vi "IniEVEScrew.vi"(8 "error in":errorcluster, 10 "Screw section":string="Info", 11 "INI file path":path=path "D:/ZDX201 塗膠螺絲鎖固自動化_鴻海/ZDX201_LabView/iniData/screw_iniData.ini") -> (0 "L_file":string, 1 "R_file":string, 2 "螺絲高度LL":dbl, 3 "螺絲高度UL":dbl, 4 "txt path":path, 5 "自動運行":bool, 6 "分析計算時間":u32, 7 "offset":dbl=2.4009)   [LabVIEW 2019]
uses:
  <vilib>/Utility/config.llb/Read Key (Double).vi
  <vilib>/Utility/config.llb/Read Key (Path).vi
  <vilib>/Utility/config.llb/Read Key (String).vi
  <vilib>/Utility/config.llb/Read Key (Boolean).vi
  <vilib>/Utility/config.llb/Read Key (U32).vi
  <vilib>/Utility/config.llb/NI_LVConfig.lvlib
panel:
  out "error out":errorcluster
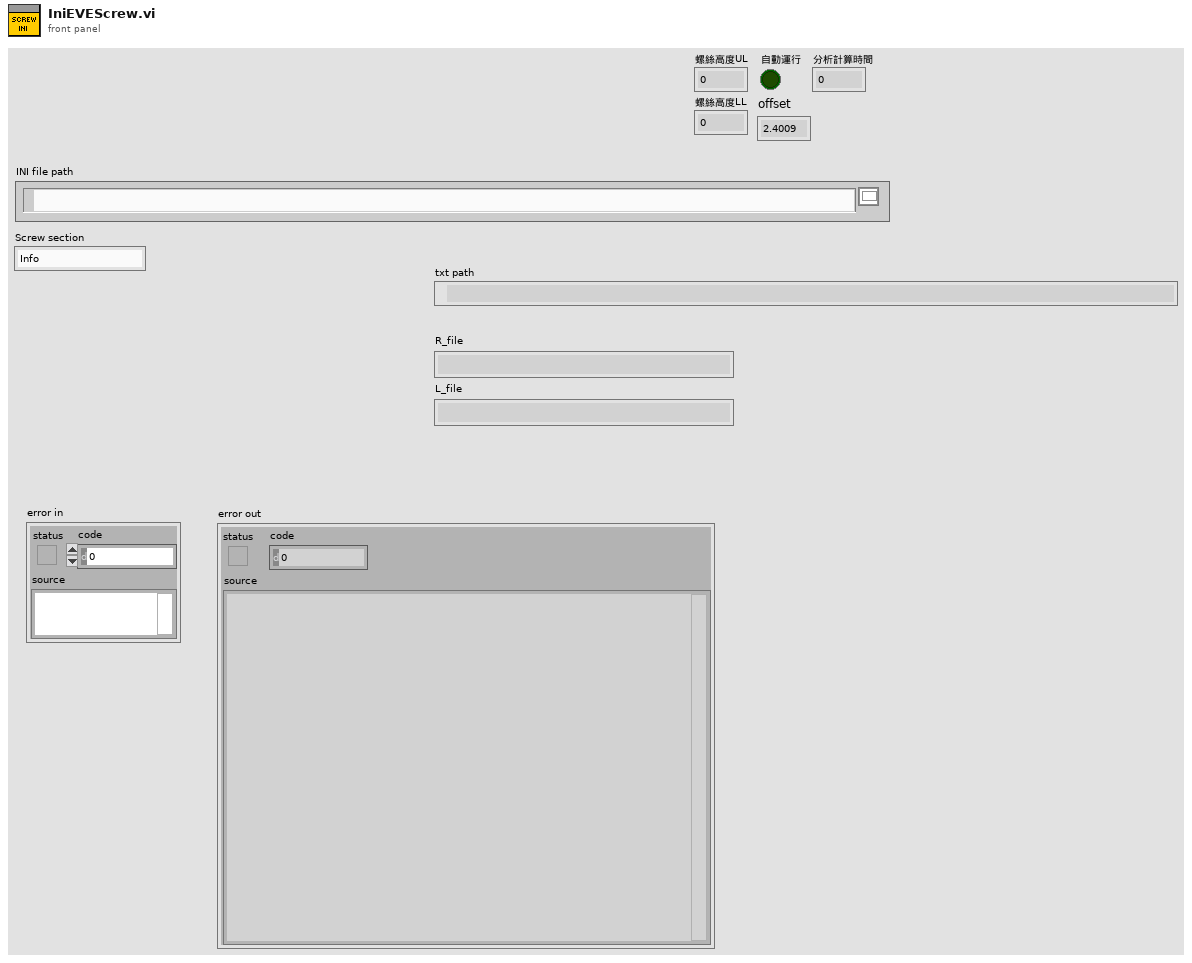
[diagram p1: front panel]
types:
  T1 = typedef "NI_LVConfig.lvlib/Config Data RefNum.ctl" = refnum<k1>
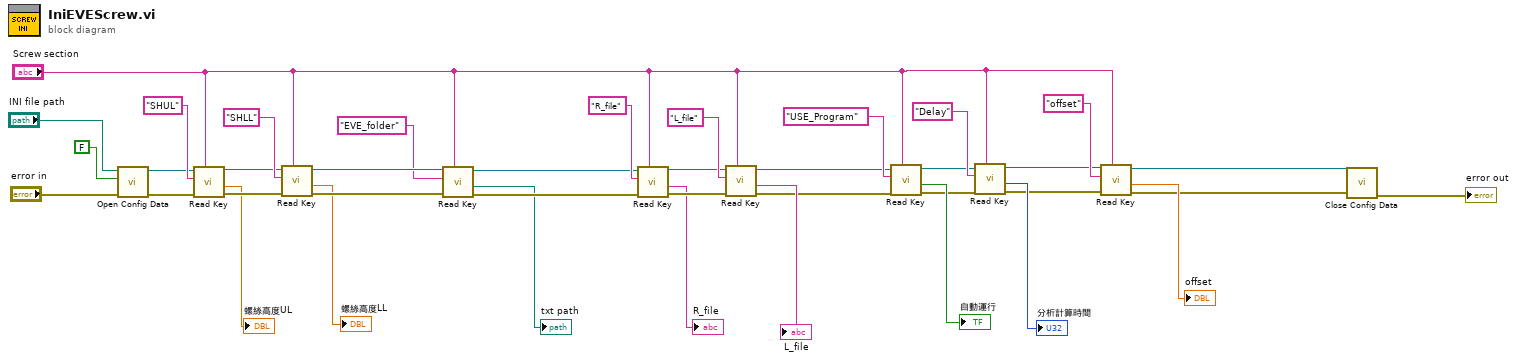
[diagram p0: block diagram]
diagram:
  n1 = call <vilib>:"Open Config Data.vi"("error in (no error)"="error in", "create file if necessary (T)"=FALSE ("create file if necessary? (T)"), "configuration file path"="INI file path") -> ("error out"=w37:errorcluster, "refnum"=w35:T1)  [unwired: 6 in, 1 out]
  n2 = call-poly <vilib>:"Read Key.vi"("section"="Screw section", "error in (no error)"=w37, "key"="SHUL", "refnum"=w35) -> ("error out"=w30:errorcluster, "value"=→"螺絲高度UL":dbl, "refnum out"=w31:T1)  [unwired: 1 in, 4 out]
  n3 = call-poly <vilib>:"Read Key.vi"("section"="Screw section", "error in (no error)"=w30, "key"="SHLL", "refnum"=w31) -> ("error out"=w23:errorcluster, "value"=→"螺絲高度LL":dbl, "refnum out"=w24:T1)  [unwired: 1 in, 4 out]
  n4 = call-poly <vilib>:"Read Key.vi"("section"="Screw section", "error in (no error)"=w23, "key"="EVE_folder", "refnum"=w24) -> ("error out"=w21:errorcluster, "value"=→"txt path":path, "refnum out"=w20:T1)  [unwired: 1 in, 4 out]
  n5 = call-poly <vilib>:"Read Key.vi"("section"="Screw section", "error in (no error)"=w21, "key"="R_file", "refnum"=w20) -> ("error out"=w26:errorcluster, "value"=→"R_file":string, "refnum out"=w27:T1)  [unwired: 2 in, 3 out]
  n6 = call-poly <vilib>:"Read Key.vi"("section"="Screw section", "error in (no error)"=w26, "key"="L_file", "refnum"=w27) -> ("error out"=w14:errorcluster, "value"=→"L_file":string, "refnum out"=w15:T1)  [unwired: 2 in, 3 out]
  n7 = call-poly <vilib>:"Read Key.vi"("section"="Screw section", "error in (no error)"=w14, "key"="USE_Program", "refnum"=w15) -> ("error out"=w10:errorcluster, "value"=→"自動運行":bool, "refnum out"=w11:T1)  [unwired: 1 in, 4 out]
  n8 = call-poly <vilib>:"Read Key.vi"("section"="Screw section", "error in (no error)"=w10, "key"="Delay", "refnum"=w11) -> ("error out"=w5:errorcluster, "value"=→"分析計算時間":u32, "refnum out"=w7:T1)  [unwired: 1 in, 4 out]
  n9 = call-poly <vilib>:"Read Key.vi"("section"="Screw section", "error in (no error)"=w5, "key"="offset", "refnum"=w7) -> ("error out"=w2:errorcluster, "value"=→"offset":dbl, "refnum out"=w3:T1)  [unwired: 1 in, 4 out]
  n10 = call <vilib>:"Close Config Data.vi"("error in (no error)"=w2, "refnum"=w3) -> ("error out"=→"error out":errorcluster)  [unwired: 1 in, 8 out]
